vi "消息推送.vi"(8 "error in (no error)":errorcluster caption="错误输入（无错误）", 9 "分析":string="1、建议排查管路是否异常\n2、供电情况是否正常", 10 "内容":string="故障告警", 11 "站点":string="测试点") -> (0 "error out":errorcluster caption="错误输出")   [LabVIEW 2016, in "Alarm interface.lvlib" / "wxpusher.lvlib"]
uses:
  wxpusher.lvlib
panel:
  out "GBK":string
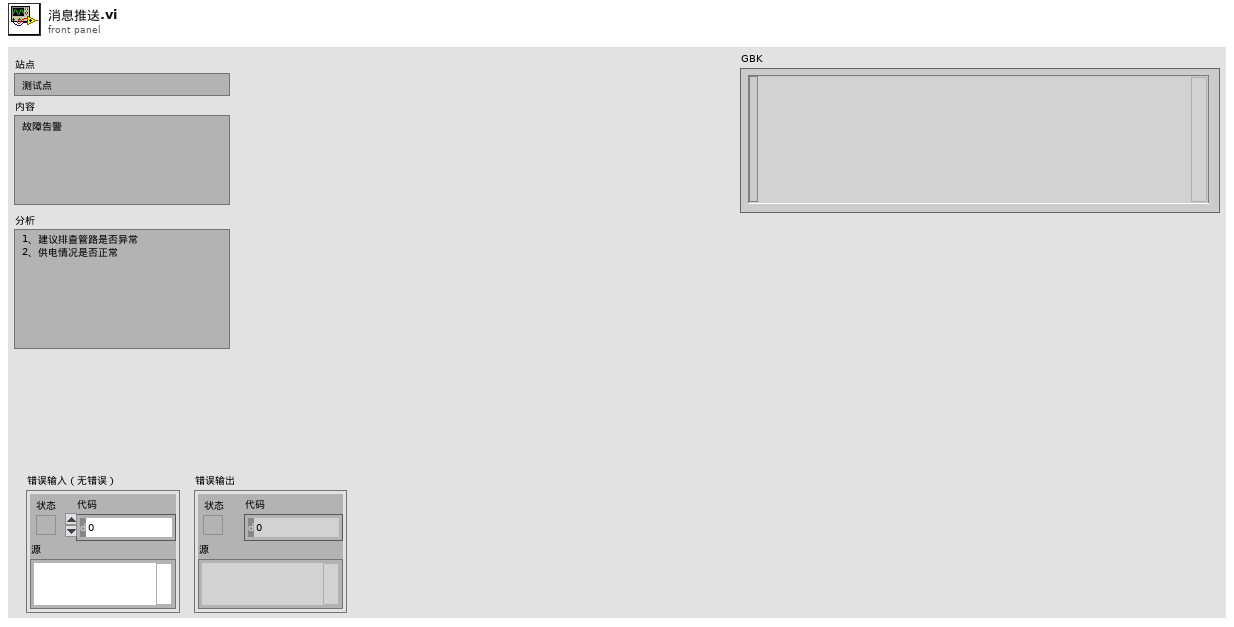
[diagram p1: front panel]
types:
  T1 = cluster{"action":string, "data":cluster{"appKey":string, "appName":string, "source":string, "time":u64, "uid":string, "userHeadImg":string, "userName":string, "extra":string}}[]
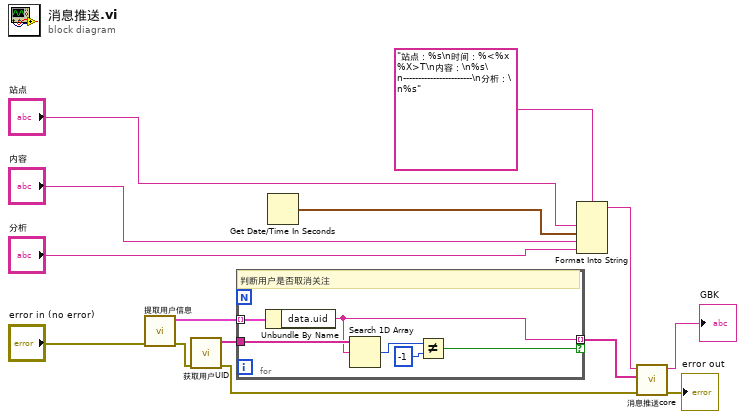
[diagram p0: block diagram]
diagram:
  n1 = call "提取用户信息.vi"("error in (no error)"="error in (no error)") -> ("error out"=w5:errorcluster, "用户信息"=w14:T1)  [unwired: 9 in]
  n2 = call "获取用户UID.vi"("error in (no error)"=w5) -> ("error out"=w3:errorcluster, "uid"=w4:string[])  [unwired: 9 in]
  n3 = for {
    tunnel: w14 -> [w20] mode=indexing
    tunnel: [w18] -> w13 mode=indexing if=w15
    tunnel: w4 -> [w19]
    # "判断用户是否取消关注"
    n4 = Unbundle By Name(w20) -> ("data.uid"=w18:string)
    n5 = Search 1D Array(1D array=w19, element=w18) -> (index of element=w17:i32)  [unwired: 1 in]
    n6 = Not Equal?(x=w17, y=-1) -> (x != y?=w15:bool)
  }
  n7 = Get Date/Time In Seconds() -> (seconds since 1Jan1904=w11:timestamp)
  n8 = Format Into String(format string="站点：%s\n时间：%<%x %X>T\n内容：\n%s\n-----------------------\n分析：\n%s" ("格式字符串"), "站点", w11, "内容", "分析") -> (resulting string=w7:string)  [unwired: 2 in, 1 out]
  n9 = call "消息推送core.vi"("error in (no error)"=w3, "数组"=w13, "content"=w7) -> ("error out"=→"error out":errorcluster, "GBK"=→"GBK":string)  [unwired: 7 in]
